vi "Modbus Status Bitmap System Status.vi"(7 "isGenOn":bool[](array[boolean]), 8 "Error In":errorcluster, 9 "FPGA Data In":T3 {"SSG Active Current" format="%2.1f"; "PV Reactive Power (L1)" format="%2.1f"; "PV Reactive Power (L2)" format="%2.1f"; "PV Total Reactive Power" format="%2.1f"; "Gen Reactive Power (L1)" format="%2.1f"; "Gen Reactive Power (L2)" format="%2.1f"; "Gen Total Reactive Power" format="%2.1f"; "SSG Reactive Power (L1)" format="%2.1f"; "SSG Reactive Power (L2)" format="%2.1f"; "SSG Total Reactive Power" format="%2.1f"; "PV Total Current" format="%2.1f"; "PV Total Voltage" format="%2.1f"; "PV Active Power (L1)" format="%2.1f"; "PV Active Power (L2)" format="%2.1f"; "PV App Power (L1)" format="%2.1f"; "PV App Power (L2)" format="%2.1f"; "PV Total Active Power" format="%2.1f"; "PV Total App Power" format="%2.1f"; "PV Arms (L1)" format="%2.1f"; "PV Arms (L2)" format="%2.1f"; "PV Vrms (L1)" format="%2.1f"; "PV Vrms (L2)" format="%2.1f"; "Gen Total Current" format="%2.1f"; "SSG Total Current" format="%2.1f"; "Gen Total Voltage" format="%2.1f"; "SSG Total Voltage" format="%2.1f"; "Gen Active Power (L1)" format="%2.1f"; "Gen Active Power (L2)" format="%2.1f"; "SSG Active Power (L1)" format="%2.1f"; "SSG Active Power (L2)" format="%2.1f"; "Gen App Power (L1)" format="%2.1f"; "Gen App Power (L2)" format="%2.1f"; "SSG App Power (L1)" format="%2.1f"; "SSG App Power (L2)" format="%2.1f"; "Gen Total Active Power" format="%2.1f"; "Gen Total App Power" format="%2.1f"; "Gen Arms (L1)" format="%2.1f"; "Gen Arms (L2)" format="%2.1f"; "Gen Vrms (L1)" format="%2.1f"; "Gen Vrms (L2)" format="%2.1f"; "SSG Total Active Power" format="%2.1f"; "SSG Total App Power" format="%2.1f"; "SSG Arms (L1)" format="%2.1f"; "SSG Arms (L2)" format="%2.1f"; "SSG Vrms (L1)" format="%2.1f"; "SSG Vrms (L2)" format="%2.1f"}, 10 "Gen Data Array":T2[](array[typedef]) {"TotalFuel(L)" format="%.2f"; "FuelRate(L/H)" format="%.2f"; "ApparentPower(VA)" format="%.2f"; "BattVoltage(V)" format="%.2f"; "Freq(Hz)" format="%.2f"; "RunHours(hr)" format="%.2f"; "PowerFactor" format="%.2f"; "ReactivePower(VAR)" format="%.2f"; "ActivePower(W)" format="%.2f"}, 11 "Real Time State":T1) -> (0 "Error Out":errorcluster, 3 "System Status":i16)   [LabVIEW 2014]
uses:
  Controls/FPGA Data.ctl
  Controls/Gen Data.ctl
  Controls/RT State.ctl
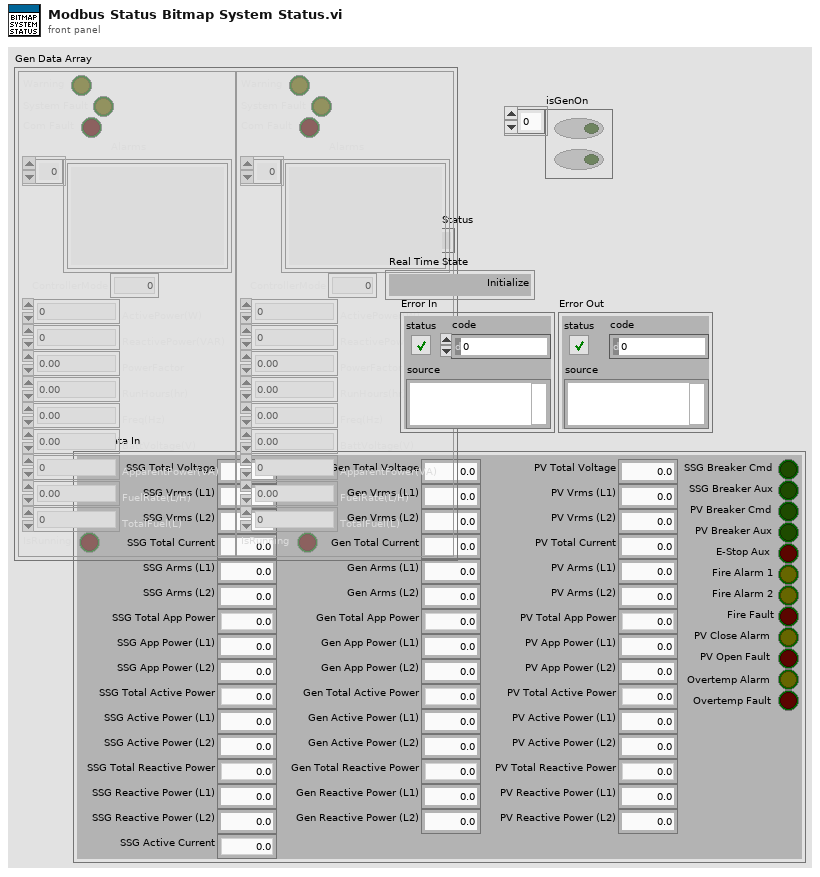
[diagram p1: front panel]
types:
  T1 = typedef "RT State.ctl" = enum16{"Initialize", "Ready", "Startup 1 - Start Genset", "Startup 2 - Start Inverter", "Startup 3 - Battery Match", "SpotGen - Start", "SpotGen - Charge", "SpotGen - Desync", "SpotGen - Discharge", "SpotGen - Sync", "Shutdown", "INVALID STATE"}
  T2 = typedef "Gen Data.ctl" = cluster{"Warning":bool, "System Fault":bool, "Com Fault":bool, "Alarms":string[], "ControllerMode":u16, "ActivePower(W)":i32, "ReactivePower(VAR)":i32, "PowerFactor":dbl, "RunHours(hr)":dbl, "Freq(Hz)":dbl, "BattVoltage(V)":dbl, "ApparentPower(VA)":i32, "FuelRate(L/H)":dbl, "TotalFuel(L)":u32, "IsRunning":bool}
  T3 = typedef "FPGA Data.ctl" = cluster{"Gen Total Voltage":dbl, "Gen Vrms (L1)":dbl, "Gen Vrms (L2)":dbl, "Gen Total Current":dbl, "Gen Arms (L1)":dbl, "Gen Arms (L2)":dbl, "Gen Total App Power":dbl, "Gen App Power (L1)":dbl, "Gen App Power (L2)":dbl, "Gen Total Active Power":dbl, "Gen Active Power (L1)":dbl, "Gen Active Power (L2)":dbl, "Gen Total Reactive Power":dbl, "Gen Reactive Power (L1)":dbl, "Gen Reactive Power (L2)":dbl, "SSG Total Voltage":dbl, "SSG Vrms (L1)":dbl, "SSG Vrms (L2)":dbl, "SSG Total Current":dbl, "SSG Arms (L1)":dbl, "SSG Arms (L2)":dbl, "SSG Total App Power":dbl, "SSG App Power (L1)":dbl, "SSG App Power (L2)":dbl, "SSG Total Active Power":dbl, "SSG Active Power (L1)":dbl, "SSG Active Power (L2)":dbl, "SSG Total Reactive Power":dbl, "SSG Reactive Power (L1)":dbl, "SSG Reactive Power (L2)":dbl, "PV Total Voltage":dbl, "PV Vrms (L1)":dbl, "PV Vrms (L2)":dbl, "PV Total Current":dbl, "PV Arms (L1)":dbl, "PV Arms (L2)":dbl, "PV Total App Power":dbl, "PV App Power (L1)":dbl, "PV App Power (L2)":dbl, "PV Total Active Power":dbl, "PV Active Power (L1)":dbl, "PV Active Power (L2)":dbl, "PV Total Reactive Power":dbl, "PV Reactive Power (L1)":dbl, "PV Reactive Power (L2)":dbl, "SSG Breaker Cmd":bool, "SSG Breaker Aux":bool, "PV Breaker Cmd":bool, "PV Breaker Aux":bool, "E-Stop Aux":bool, "Fire Alarm 1":bool, "Fire Alarm 2":bool, "Fire Fault":bool, "PV Close Alarm":bool, "SSG Active Current":dbl, "Overtemp Alarm":bool, "Overtemp Fault":bool, "PV Open Fault":bool}
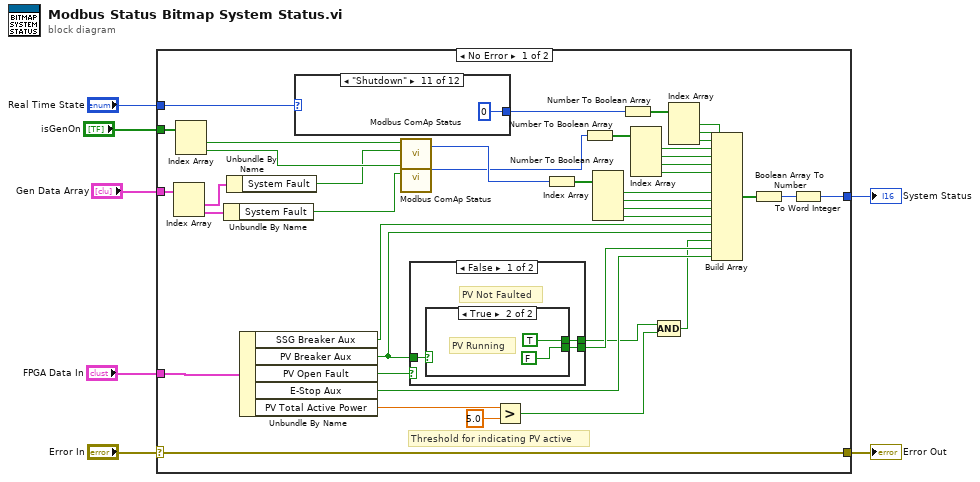
[diagram p0: block diagram]
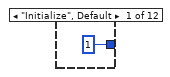
[diagram p2: hidden frame]
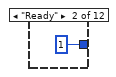
[diagram p3: hidden frame]
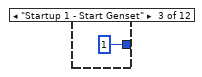
[diagram p4: hidden frame]
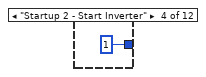
[diagram p5: hidden frame]
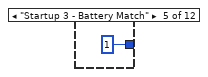
[diagram p6: hidden frame]
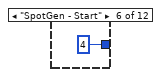
[diagram p7: hidden frame]
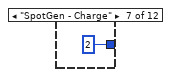
[diagram p8: hidden frame]
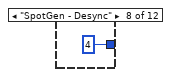
[diagram p9: hidden frame]
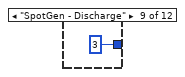
[diagram p10: hidden frame]
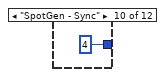
[diagram p11: hidden frame]
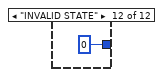
[diagram p12: hidden frame]
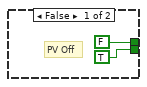
[diagram p13: hidden frame]
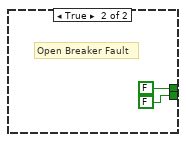
[diagram p14: hidden frame]
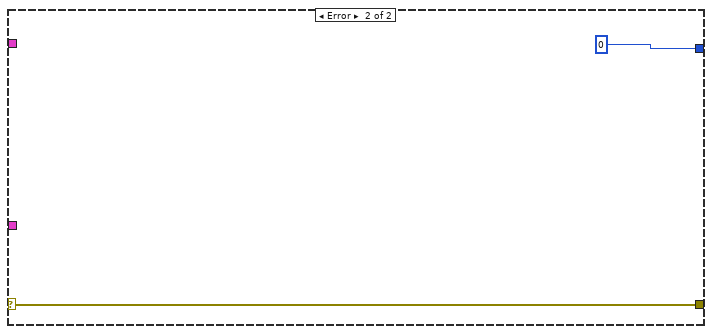
[diagram p15: hidden frame]
diagram:
  n1 = case shown="No Error" "Error In" {
    selector: "Error In" -> [w27 w71]
    tunnel: "FPGA Data In" -> [w30 _]
    tunnel: [w28 i16 0] -> w6
    tunnel: [w27 w71] -> w4
    tunnel: "Gen Data Array" -> [w26 _]
    tunnel: "Real Time State" -> [w23 _]
    tunnel: "isGenOn" -> [w12 _]
    frame No Error {
      # "Threshold for indicating PV active"
      n2 = Index Array(array=w26) -> (element #1=w25:T2, element #2=w24:T2)  [unwired: 2 in]
      n3 = Index Array(array=w12) -> (element #1=w11:bool, element #2=w10:bool)  [unwired: 2 in]
      n4 = Unbundle By Name(w24) -> ("System Fault"=w8:bool)
      n5 = Unbundle By Name(w25) -> ("System Fault"=w9:bool)
      n6 = Unbundle By Name(w30) -> ("SSG Breaker Aux"=w18:bool, "PV Breaker Aux"=w19:bool, "PV Open Fault"=w31:bool, "E-Stop Aux"=w33:bool, "PV Total Active Power"=w17:dbl)
      n7 = case shown="\"Shutdown\"" w23 {
        tunnel: [u32 1 ("number") u32 1 ("number") u32 1 ("number") u32 1 ("number") u32 1 ("number") u32 4 ("number") u32 2 ("number") u32 4 ("number") u32 3 ("number") u32 4 ("number") u32 0 ("number") u32 0 ("number")] -> w22
        frame "Initialize", Default {
        }
        frame "Ready" {
        }
        frame "Startup 1 - Start Genset" {
        }
        frame "Startup 2 - Start Inverter" {
        }
        frame "Startup 3 - Battery Match" {
        }
        frame "SpotGen - Start" {
        }
        frame "SpotGen - Charge" {
        }
        frame "SpotGen - Desync" {
        }
        frame "SpotGen - Discharge" {
        }
        frame "SpotGen - Sync" {
        }
        frame "Shutdown" {
        }
        frame "INVALID STATE" {
        }
      }
      n8 = call "Modbus ComAp Status.vi"("IsGenOn"=w11, "Alarm"=w9) -> ("Status Out"=w21:u16)  [unwired: 4 in]
      n9 = call "Modbus ComAp Status.vi"("IsGenOn"=w10, "Alarm"=w8) -> ("Status Out"=w20:u16)  [unwired: 4 in]
      n10 = case shown="False" w31 {
        tunnel: [w62 FALSE] -> w15
        tunnel: [w61 FALSE] -> w32
        tunnel: w19 -> [w63 _]
        frame False {
          # "PV Not Faulted"
          n11 = case shown="True" w63 {
            tunnel: [FALSE TRUE] -> w62
            tunnel: [TRUE FALSE] -> w61
            frame False {
              # "PV Off"
            }
            frame True {
              # "PV Running"
            }
          }
        }
        frame True {
          # "Open Breaker Fault"
        }
      }
      n12 = Greater?(x=w17, y=5.0) -> (0:w13:bool)
      n13 = Number To Boolean Array(number=w21) -> (Boolean array=w42:bool[])
      n14 = Number To Boolean Array(number=w20) -> (Boolean array=w43:bool[])
      n15 = Index Array(array=w42) -> (element #1=w37:bool, element #2=w36:bool, element #3=w35:bool, element #4=w34:bool)  [unwired: 4 in]
      n16 = Number To Boolean Array(number=w22) -> (Boolean array=w48:bool[])
      n17 = Index Array(array=w43) -> (element #1=w41:bool, element #2=w40:bool, element #3=w39:bool, element #4=w38:bool)  [unwired: 4 in]
      n18 = Compound Arithmetic op=AND(w15, w13) -> (w14:bool)
      n19 = Index Array(array=w48) -> (element #1=w47:bool, element #2=w46:bool, element #3=w45:bool)  [unwired: 3 in]
      n20 = Build Array(w47, w46, w45, w41, w40, w39, w38, w37, w36, w35, w34, w18, w19, w14, w32, w33) -> (w44:bool[])
      n21 = Boolean Array To Number(Boolean array=w44) -> (number=w29:u32)
      n22 = To Word Integer(number=w29) -> (16bit integer=w28:i16)
    }
    frame Error {
    }
  }
  "System Status" <- w6
  "Error Out" <- w4
